vi "Switch0102_DataLog.vi"() -> ()   [LabVIEW 2016]
panel:
  in  "Start 3":bool=TRUE
  out "error out 2":errorcluster
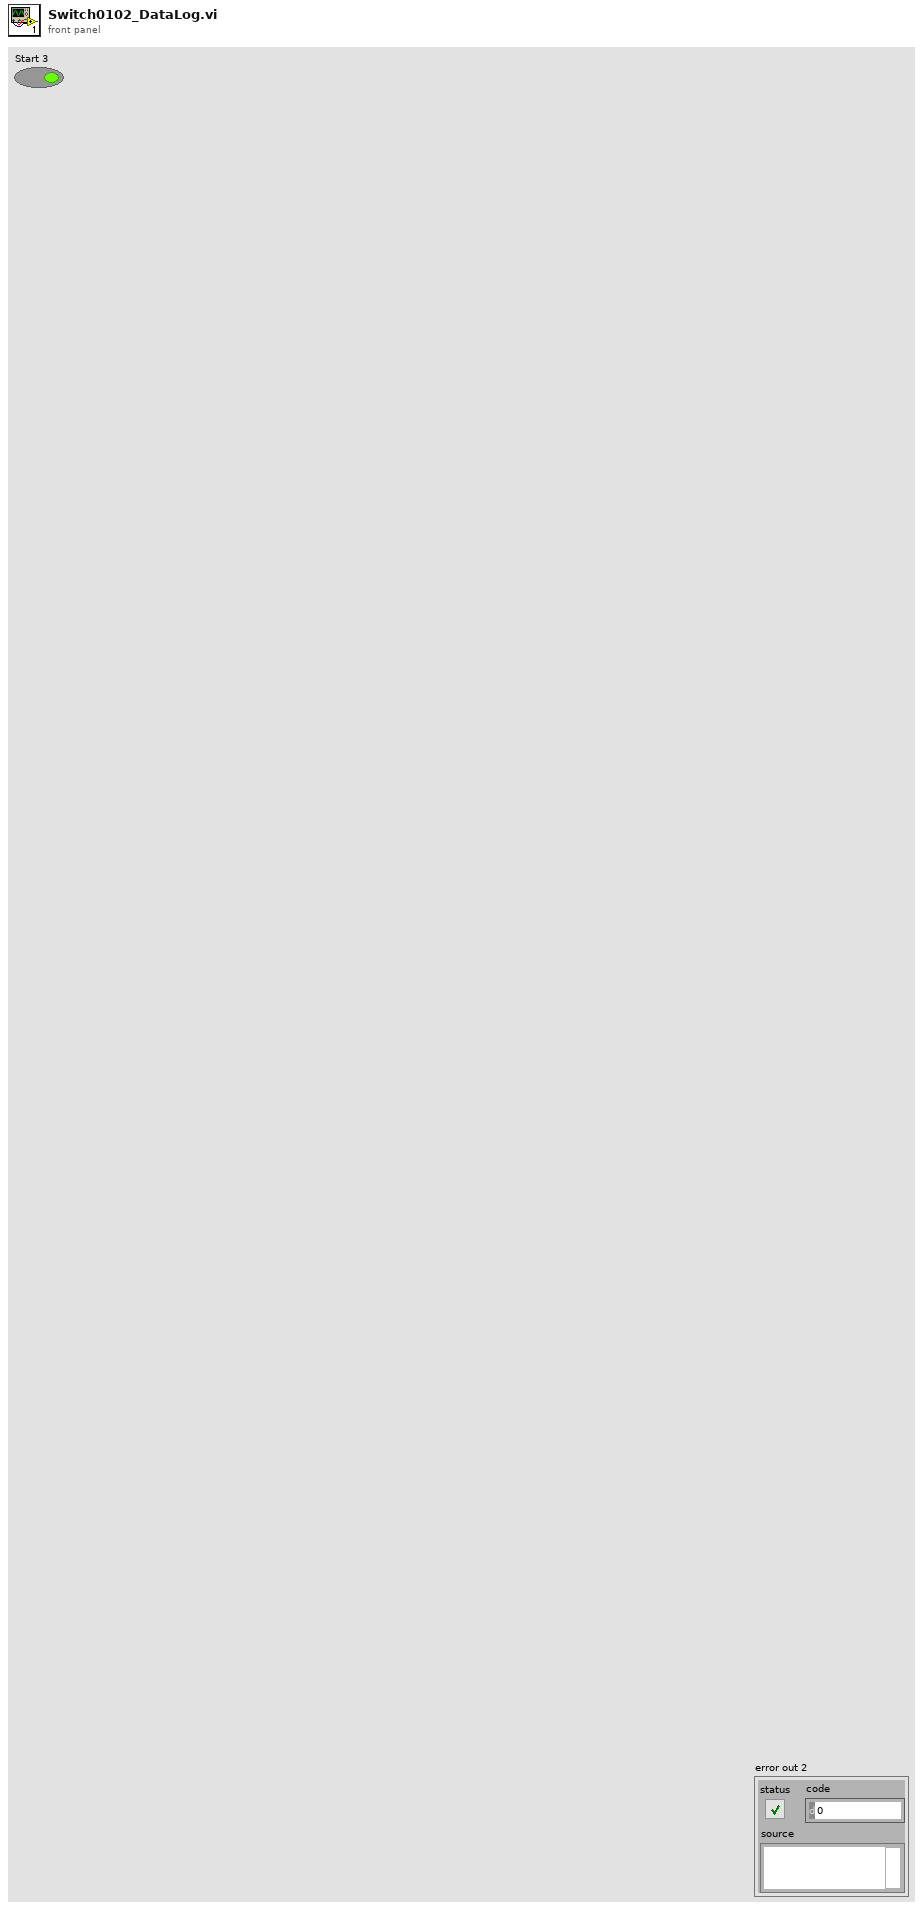
[diagram p1: front panel]
types:
  T1 = enum16{"open", "open or create", "create or replace", "create", "open (read-only)"}
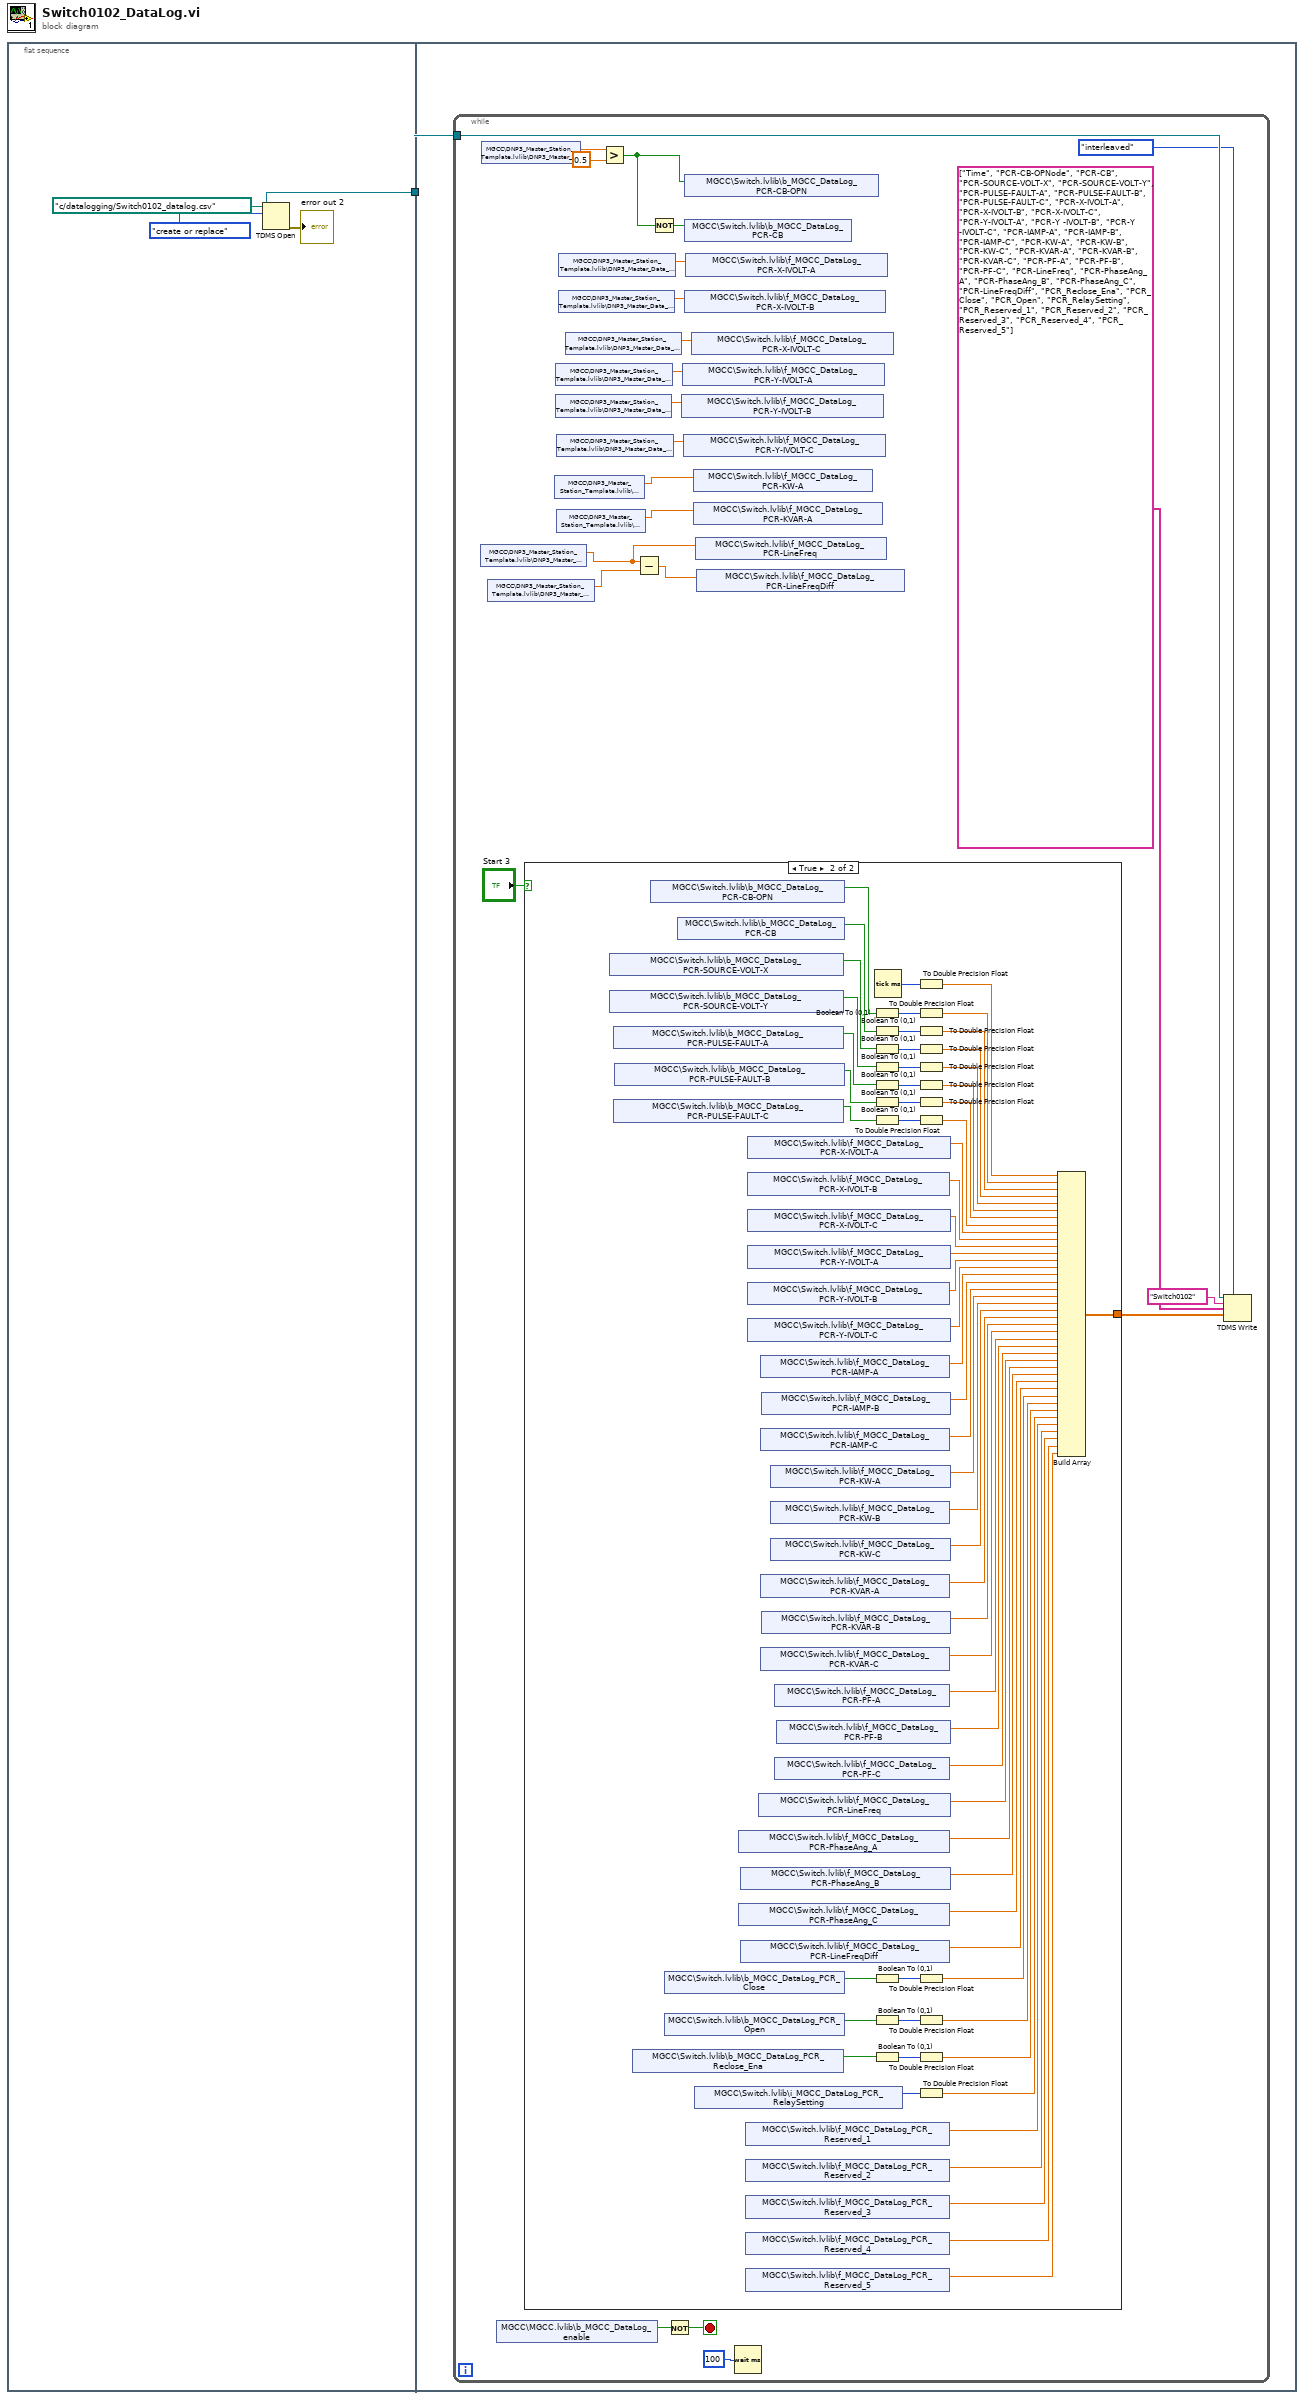
[diagram p0: block diagram]
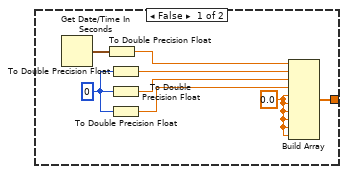
[diagram p2: hidden frame]
diagram:
  n1 = flat-sequence {
    tunnel: [w4] -> w1
    tunnel: w1 -> [w6]
    frame #0 {
      n2 = TDMS Open(10:T1."create or replace" ("operation (0:open)"), 11:path "c:/datalogging/Switch0102_datalog.csv" ("file path (dialog if empty)")) -> (0:→"error out 2":errorcluster, 3:w4:refnum<k34>)  [unwired: 5 in]
    }
    frame #1 {
      n3 = while {
        tunnel: w6 -> [w28]
        stop <- w22 stop-if-true
        n4 = shared-variable "MGCC\\DNP3_Master_Station_Template.lvlib\\DNP3_Master_Data_Variables.lvlib\\MS_Analog_Status.lvlib\\S0102-FREQ-L"() -> (w9:dbl)  [unwired: 1 in, 1 out]
        n5 = shared-variable "MGCC\\DNP3_Master_Station_Template.lvlib\\DNP3_Master_Data_Variables.lvlib\\MS_Analog_Status.lvlib\\S0102-status"() -> (w21:dbl)  [unwired: 1 in, 1 out]
        n6 = shared-variable "MGCC\\DNP3_Master_Station_Template.lvlib\\DNP3_Master_Data_Variables.lvlib\\MS_Analog_Status.lvlib\\S0102-FREQ-R"() -> (w11:dbl)  [unwired: 1 in, 1 out]
        n7 = shared-variable "MGCC\\MGCC.lvlib\\b_MGCC_DataLog_enable"() -> (w23:bool)  [unwired: 1 in, 1 out]
        n8 = case shown="True" "Start 3" {
          tunnel: [w33 w79] -> w26
          frame False {
            w35 = 0.0
            w32 = 0
            n9 = Get Date/Time In Seconds() -> (seconds since 1Jan1904=w31:timestamp)
            n10 = To Double Precision Float(number=w31) -> (double precision float=w34:dbl)
            n11 = To Double Precision Float(number=w32) -> (double precision float=w38:dbl)
            n12 = To Double Precision Float(number=w32) -> (double precision float=w37:dbl)
            n13 = To Double Precision Float(number=w32) -> (double precision float=w36:dbl)
            n14 = Build Array(w34, w38, w37, w36, w35, w35, w35, w35, w35, w35) -> (w33:dbl[])
          }
          frame True {
            n15 = shared-variable "MGCC\\Switch.lvlib\\b_MGCC_DataLog_PCR-SOURCE-VOLT-X"() -> (w99:bool)  [unwired: 1 in, 1 out]
            n16 = shared-variable "MGCC\\Switch.lvlib\\b_MGCC_DataLog_PCR-SOURCE-VOLT-Y"() -> (w98:bool)  [unwired: 1 in, 1 out]
            n17 = shared-variable "MGCC\\Switch.lvlib\\b_MGCC_DataLog_PCR-PULSE-FAULT-A"() -> (w97:bool)  [unwired: 1 in, 1 out]
            n18 = shared-variable "MGCC\\Switch.lvlib\\b_MGCC_DataLog_PCR-PULSE-FAULT-C"() -> (w95:bool)  [unwired: 1 in, 1 out]
            n19 = shared-variable "MGCC\\Switch.lvlib\\b_MGCC_DataLog_PCR-PULSE-FAULT-B"() -> (w96:bool)  [unwired: 1 in, 1 out]
            n20 = shared-variable "MGCC\\Switch.lvlib\\b_MGCC_DataLog_PCR_Reclose_Ena"() -> (w82:bool)  [unwired: 1 in, 1 out]
            n21 = shared-variable "MGCC\\Switch.lvlib\\b_MGCC_DataLog_PCR-CB-OPN"() -> (w101:bool)  [unwired: 1 in, 1 out]
            n22 = shared-variable "MGCC\\Switch.lvlib\\b_MGCC_DataLog_PCR_Close"() -> (w86:bool)  [unwired: 1 in, 1 out]
            n23 = shared-variable "MGCC\\Switch.lvlib\\b_MGCC_DataLog_PCR_Open"() -> (w84:bool)  [unwired: 1 in, 1 out]
            n24 = shared-variable "MGCC\\Switch.lvlib\\b_MGCC_DataLog_PCR-CB"() -> (w100:bool)  [unwired: 1 in, 1 out]
            n25 = shared-variable "MGCC\\Switch.lvlib\\i_MGCC_DataLog_PCR_RelaySetting"() -> (w80:i16)  [unwired: 1 in, 1 out]
            n26 = shared-variable "MGCC\\Switch.lvlib\\f_MGCC_DataLog_PCR-PhaseAng_A"() -> (w51:dbl)  [unwired: 1 in, 1 out]
            n27 = shared-variable "MGCC\\Switch.lvlib\\f_MGCC_DataLog_PCR-PhaseAng_C"() -> (w49:dbl)  [unwired: 1 in, 1 out]
            n28 = shared-variable "MGCC\\Switch.lvlib\\f_MGCC_DataLog_PCR-PhaseAng_B"() -> (w50:dbl)  [unwired: 1 in, 1 out]
            n29 = shared-variable "MGCC\\Switch.lvlib\\f_MGCC_DataLog_PCR-LineFreqDiff"() -> (w48:dbl)  [unwired: 1 in, 1 out]
            n30 = shared-variable "MGCC\\Switch.lvlib\\f_MGCC_DataLog_PCR_Reserved_1"() -> (w43:dbl)  [unwired: 1 in, 1 out]
            n31 = shared-variable "MGCC\\Switch.lvlib\\f_MGCC_DataLog_PCR_Reserved_2"() -> (w42:dbl)  [unwired: 1 in, 1 out]
            n32 = shared-variable "MGCC\\Switch.lvlib\\f_MGCC_DataLog_PCR_Reserved_3"() -> (w41:dbl)  [unwired: 1 in, 1 out]
            n33 = shared-variable "MGCC\\Switch.lvlib\\f_MGCC_DataLog_PCR_Reserved_4"() -> (w40:dbl)  [unwired: 1 in, 1 out]
            n34 = shared-variable "MGCC\\Switch.lvlib\\f_MGCC_DataLog_PCR_Reserved_5"() -> (w39:dbl)  [unwired: 1 in, 1 out]
            n35 = shared-variable "MGCC\\Switch.lvlib\\f_MGCC_DataLog_PCR-X-IVOLT-A"() -> (w70:dbl)  [unwired: 1 in, 1 out]
            n36 = shared-variable "MGCC\\Switch.lvlib\\f_MGCC_DataLog_PCR-X-IVOLT-B"() -> (w69:dbl)  [unwired: 1 in, 1 out]
            n37 = shared-variable "MGCC\\Switch.lvlib\\f_MGCC_DataLog_PCR-X-IVOLT-C"() -> (w68:dbl)  [unwired: 1 in, 1 out]
            n38 = shared-variable "MGCC\\Switch.lvlib\\f_MGCC_DataLog_PCR-Y-IVOLT-A"() -> (w67:dbl)  [unwired: 1 in, 1 out]
            n39 = shared-variable "MGCC\\Switch.lvlib\\f_MGCC_DataLog_PCR-Y-IVOLT-B"() -> (w66:dbl)  [unwired: 1 in, 1 out]
            n40 = shared-variable "MGCC\\Switch.lvlib\\f_MGCC_DataLog_PCR-Y-IVOLT-C"() -> (w65:dbl)  [unwired: 1 in, 1 out]
            n41 = shared-variable "MGCC\\Switch.lvlib\\f_MGCC_DataLog_PCR-LineFreq"() -> (w52:dbl)  [unwired: 1 in, 1 out]
            n42 = shared-variable "MGCC\\Switch.lvlib\\f_MGCC_DataLog_PCR-IAMP-A"() -> (w64:dbl)  [unwired: 1 in, 1 out]
            n43 = shared-variable "MGCC\\Switch.lvlib\\f_MGCC_DataLog_PCR-IAMP-C"() -> (w62:dbl)  [unwired: 1 in, 1 out]
            n44 = shared-variable "MGCC\\Switch.lvlib\\f_MGCC_DataLog_PCR-KVAR-A"() -> (w58:dbl)  [unwired: 1 in, 1 out]
            n45 = shared-variable "MGCC\\Switch.lvlib\\f_MGCC_DataLog_PCR-KVAR-C"() -> (w56:dbl)  [unwired: 1 in, 1 out]
            n46 = shared-variable "MGCC\\Switch.lvlib\\f_MGCC_DataLog_PCR-IAMP-B"() -> (w63:dbl)  [unwired: 1 in, 1 out]
            n47 = shared-variable "MGCC\\Switch.lvlib\\f_MGCC_DataLog_PCR-KVAR-B"() -> (w57:dbl)  [unwired: 1 in, 1 out]
            n48 = shared-variable "MGCC\\Switch.lvlib\\f_MGCC_DataLog_PCR-KW-A"() -> (w61:dbl)  [unwired: 1 in, 1 out]
            n49 = shared-variable "MGCC\\Switch.lvlib\\f_MGCC_DataLog_PCR-KW-B"() -> (w60:dbl)  [unwired: 1 in, 1 out]
            n50 = shared-variable "MGCC\\Switch.lvlib\\f_MGCC_DataLog_PCR-KW-C"() -> (w59:dbl)  [unwired: 1 in, 1 out]
            n51 = shared-variable "MGCC\\Switch.lvlib\\f_MGCC_DataLog_PCR-PF-A"() -> (w55:dbl)  [unwired: 1 in, 1 out]
            n52 = shared-variable "MGCC\\Switch.lvlib\\f_MGCC_DataLog_PCR-PF-C"() -> (w53:dbl)  [unwired: 1 in, 1 out]
            n53 = shared-variable "MGCC\\Switch.lvlib\\f_MGCC_DataLog_PCR-PF-B"() -> (w54:dbl)  [unwired: 1 in, 1 out]
            n54 = Boolean To (0,1)(Boolean=w101) -> (0, 1=w92:i16)
            n55 = Boolean To (0,1)(Boolean=w100) -> (0, 1=w93:i16)
            n56 = Boolean To (0,1)(Boolean=w99) -> (0, 1=w87:i16)
            n57 = Boolean To (0,1)(Boolean=w98) -> (0, 1=w88:i16)
            n58 = Boolean To (0,1)(Boolean=w97) -> (0, 1=w89:i16)
            n59 = Boolean To (0,1)(Boolean=w96) -> (0, 1=w90:i16)
            n60 = Boolean To (0,1)(Boolean=w95) -> (0, 1=w91:i16)
            n61 = Boolean To (0,1)(Boolean=w86) -> (0, 1=w85:i16)
            n62 = Boolean To (0,1)(Boolean=w84) -> (0, 1=w83:i16)
            n63 = Boolean To (0,1)(Boolean=w82) -> (0, 1=w81:i16)
            n64 = Tick Count (ms)() -> (millisecond timer value=w94:u32)
            n65 = To Double Precision Float(number=w94) -> (double precision float=w78:dbl)
            n66 = To Double Precision Float(number=w92) -> (double precision float=w77:dbl)
            n67 = To Double Precision Float(number=w93) -> (double precision float=w76:dbl)
            n68 = To Double Precision Float(number=w87) -> (double precision float=w75:dbl)
            n69 = To Double Precision Float(number=w88) -> (double precision float=w74:dbl)
            n70 = To Double Precision Float(number=w89) -> (double precision float=w73:dbl)
            n71 = To Double Precision Float(number=w90) -> (double precision float=w72:dbl)
            n72 = To Double Precision Float(number=w91) -> (double precision float=w71:dbl)
            n73 = To Double Precision Float(number=w85) -> (double precision float=w47:dbl)
            n74 = To Double Precision Float(number=w83) -> (double precision float=w46:dbl)
            n75 = To Double Precision Float(number=w81) -> (double precision float=w45:dbl)
            n76 = To Double Precision Float(number=w80) -> (double precision float=w44:dbl)
            n77 = Build Array(w78, w77, w76, w75, w74, w73, w72, w71, w70, w69, w68, w67, w66, w65, w64, w63, w62, w61, w60, w59, w58, w57, w56, w55, w54, w53, w52, w51, w50, w49, w48, w47, w46, w45, w44, w43, w42, w41, w40, w39) -> (w79:dbl[])
          }
        }
        n78 = shared-variable "MGCC\\DNP3_Master_Station_Template.lvlib\\DNP3_Master_Data_Variables.lvlib\\MS_Analog_Status.lvlib\\S0102-APF"() -> (w8:dbl)  [unwired: 1 in, 1 out]
        n79 = shared-variable "MGCC\\DNP3_Master_Station_Template.lvlib\\DNP3_Master_Data_Variables.lvlib\\MS_Analog_Status.lvlib\\S0102-MAG-A-R"() -> (w14:dbl)  [unwired: 1 in, 1 out]
        n80 = shared-variable "MGCC\\DNP3_Master_Station_Template.lvlib\\DNP3_Master_Data_Variables.lvlib\\MS_Analog_Status.lvlib\\S0102-MAG-B-R"() -> (w13:dbl)  [unwired: 1 in, 1 out]
        n81 = shared-variable "MGCC\\DNP3_Master_Station_Template.lvlib\\DNP3_Master_Data_Variables.lvlib\\MS_Analog_Status.lvlib\\S0102-MAG-C-R"() -> (w12:dbl)  [unwired: 1 in, 1 out]
        n82 = shared-variable "MGCC\\DNP3_Master_Station_Template.lvlib\\DNP3_Master_Data_Variables.lvlib\\MS_Analog_Status.lvlib\\S0102-RPF"() -> (w7:dbl)  [unwired: 1 in, 1 out]
        n83 = shared-variable "MGCC\\DNP3_Master_Station_Template.lvlib\\DNP3_Master_Data_Variables.lvlib\\MS_Analog_Status.lvlib\\S0102-MAG-A-L"() -> (w17:dbl)  [unwired: 1 in, 1 out]
        n84 = shared-variable "MGCC\\DNP3_Master_Station_Template.lvlib\\DNP3_Master_Data_Variables.lvlib\\MS_Analog_Status.lvlib\\S0102-MAG-B-L"() -> (w16:dbl)  [unwired: 1 in, 1 out]
        n85 = shared-variable "MGCC\\DNP3_Master_Station_Template.lvlib\\DNP3_Master_Data_Variables.lvlib\\MS_Analog_Status.lvlib\\S0102-MAG-C-L"() -> (w15:dbl)  [unwired: 1 in, 1 out]
        n86 = Greater?(x=w21, y=0.5) -> (0:w18:bool)
        n87 = Subtract(x=w9, y=w11) -> (x-y=w10:dbl)
        n88 = Not(x=w18) -> (.not. x?=w19:bool)
        n89 = Not(x=w23) -> (.not. x?=w22:bool)
        n90 = shared-variable "MGCC\\Switch.lvlib\\f_MGCC_DataLog_PCR-Y-IVOLT-B"(w13) -> ()  [unwired: 1 in, 1 out]
        n91 = shared-variable "MGCC\\Switch.lvlib\\f_MGCC_DataLog_PCR-Y-IVOLT-A"(w14) -> ()  [unwired: 1 in, 1 out]
        n92 = shared-variable "MGCC\\Switch.lvlib\\f_MGCC_DataLog_PCR-Y-IVOLT-C"(w12) -> ()  [unwired: 1 in, 1 out]
        n93 = shared-variable "MGCC\\Switch.lvlib\\b_MGCC_DataLog_PCR-CB-OPN"(w18) -> ()  [unwired: 1 in, 1 out]
        n94 = shared-variable "MGCC\\Switch.lvlib\\b_MGCC_DataLog_PCR-CB"(w19) -> ()  [unwired: 1 in, 1 out]
        n95 = shared-variable "MGCC\\Switch.lvlib\\f_MGCC_DataLog_PCR-X-IVOLT-B"(w16) -> ()  [unwired: 1 in, 1 out]
        n96 = shared-variable "MGCC\\Switch.lvlib\\f_MGCC_DataLog_PCR-X-IVOLT-A"(w17) -> ()  [unwired: 1 in, 1 out]
        n97 = shared-variable "MGCC\\Switch.lvlib\\f_MGCC_DataLog_PCR-X-IVOLT-C"(w15) -> ()  [unwired: 1 in, 1 out]
        n98 = shared-variable "MGCC\\Switch.lvlib\\f_MGCC_DataLog_PCR-KW-A"(w8) -> ()  [unwired: 1 in, 1 out]
        n99 = shared-variable "MGCC\\Switch.lvlib\\f_MGCC_DataLog_PCR-KVAR-A"(w7) -> ()  [unwired: 1 in, 1 out]
        n100 = shared-variable "MGCC\\Switch.lvlib\\f_MGCC_DataLog_PCR-LineFreq"(w9) -> ()  [unwired: 1 in, 1 out]
        n101 = shared-variable "MGCC\\Switch.lvlib\\f_MGCC_DataLog_PCR-LineFreqDiff"(w10) -> ()  [unwired: 1 in, 1 out]
        n102 = Wait (ms)(milliseconds to wait=u32 100) -> ()  [unwired: 1 out]
        n103 = TDMS Write(0:w28, 1:enum16{"decimated", "interleaved"}."interleaved" ("data layout (0:decimated)"), 5:"Switch0102" ("group name in (Untitled)"), 7:string[] ["Time", "PCR-CB-OPNode", "PCR-CB", "PCR-SOURCE-VOLT-X", "PCR-SOURCE-VOLT-Y", "PCR-PULSE-FAULT-A", "PCR-PULSE-FAULT-B", "PCR-PULSE-FAULT-C", "PCR-X-IVOLT-A", "PCR-X-IVOLT-B", "PCR-X-IVOLT-C", "PCR-Y-IVOLT-A", "PCR-Y -IVOLT-B", "PCR-Y -IVOLT-C", "PCR-IAMP-A", "PCR-IAMP-B", "PCR-IAMP-C", "PCR-KW-A", "PCR-KW-B", "PCR-KW-C", "PCR-KVAR-A", "PCR-KVAR-B", "PCR-KVAR-C", "PCR-PF-A", "PCR-PF-B", "PCR-PF-C", "PCR-LineFreq", "PCR-PhaseAng_A", "PCR-PhaseAng_B", "PCR-PhaseAng_C", "PCR-LineFreqDiff", "PCR_Reclose_Ena", "PCR_Close", "PCR_Open", "PCR_RelaySetting", "PCR_Reserved_1", "PCR_Reserved_2", "PCR_Reserved_3", "PCR_Reserved_4", "PCR_Reserved_5"] ("channel name(s) in (Untitled)"), 9:w26) -> ()  [unwired: 1 in, 4 out]
      }
    }
  }
